vi "DCC_enable_outputs.vi"(7 "Enable Output":bool, 8 "Error In":errorcluster, 10 "Module No":i16, 11 "DLL Path":path) -> (0 "Error Out":errorcluster, 2 "Module No":i16, 3 "DLL Path":path)   [LabVIEW 2017]
doc: "The DCC_enable_outputs function is used to enable/disable outputs of the DCC module ‘mod_no’. If ‘mod_no’ = -1, the outputs on all active modules are enabled/disabled.\n\nOutputs should be disabled during connecting cables or setting up devices controlled with DCC module. Caution: Please stay alert that the function may control an external high voltage power supply or a detector that can be damaged by exceeding the maximum operation voltage or the maximum output current.\n\nIn particular, if you control a high voltage power supply, make sure that it is safe to turn on the voltage. Switching off a high voltage power supply by the function DCC_enable_outputs is not safe in terms of human safety, and disabling the outputs cannot be used to exclude hazard by the output voltage of externally connected high voltage power supplies.\n\nAugust 2018\nFrank Quadt & Stefan Smietana\ninfo@becker-hickl.com"
panel:
  # "(c) 2021 Becker & Hickl GmbH\n     All Rights Reserved."
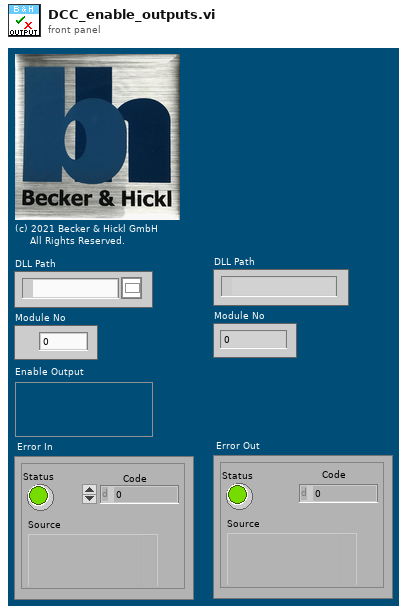
[diagram p1: front panel]
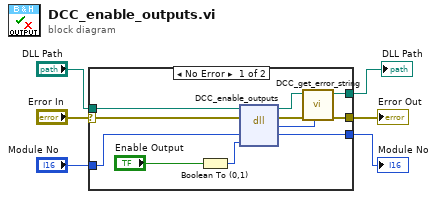
[diagram p0: block diagram]
diagram:
  n1 = case shown="No Error" "Error In" {
    selector: "Error In" -> [w17 w19]
    tunnel: [w10 w19] -> w5
    tunnel: [w9 w18] -> w4
    tunnel: "DLL Path" -> [w16 w18]
    tunnel: "Module No" -> [w14 w20]
    tunnel: [w13 w20] -> w1
    frame No Error {
      n2 = Boolean To (0,1)(Boolean="Enable Output") -> (0, 1=w15:i16)
      n3 = dll-call lib="C:/Program Files (x86)/BH/DCC/DLL/dcc64.dll" fn="DCC_enable_outputs"(path in=w16, error in=w17, "ModuleNo"=w14, "Enable"=w15) -> (path out=w11:path, error out=w12:errorcluster, "return type"=w8:i16, "ModuleNo"=w13:i16)  [unwired: 2 in]
      n4 = call "DCC_get_error_string.vi"("Error ID"=w8, "Error In"=w12, "DLL Path"=w11) -> ("Error Out"=w10:errorcluster, "DLL Path"=w9:path)  [unwired: 6 in, 1 out]
    }
    frame Error {
    }
  }
  "Error Out" <- w5
  "DLL Path" <- w4
  "Module No" <- w1
